vi "Image to Pixmap.vi"(8 "error in (no error)":errorcluster, 10 "image data":T1) -> (0 "error out":errorcluster, 2 "8-bit pixmap":u8[][](array[numeric]))   [LabVIEW 2016]
doc: "Takes image cluster and converts it to 8-bit pixmap. The 8-bit colors correspond to the pixmap drawn without any color input."
uses:
  <vilib>/picture/picture.llb/imagedata.ctl
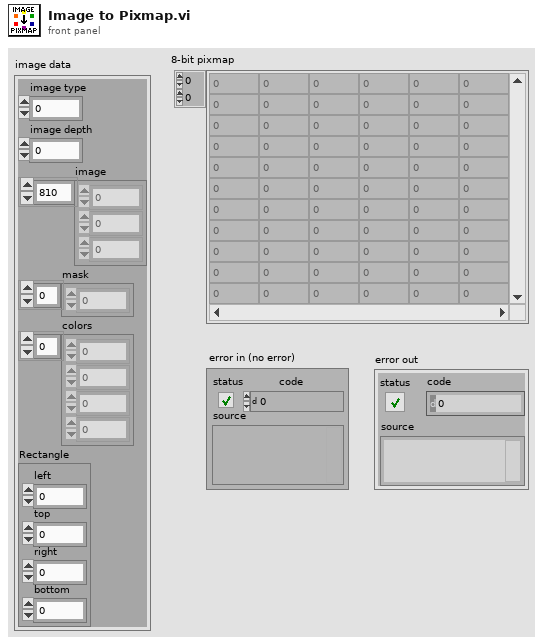
[diagram p1: front panel]
types:
  T1 = typedef "imagedata.ctl" = cluster{"image type":i32, "image depth":i32, "image":u8[], "mask":u8[], "colors":u32[], "Rectangle":cluster{"left":i16, "top":i16, "right":i16, "bottom":i16}}
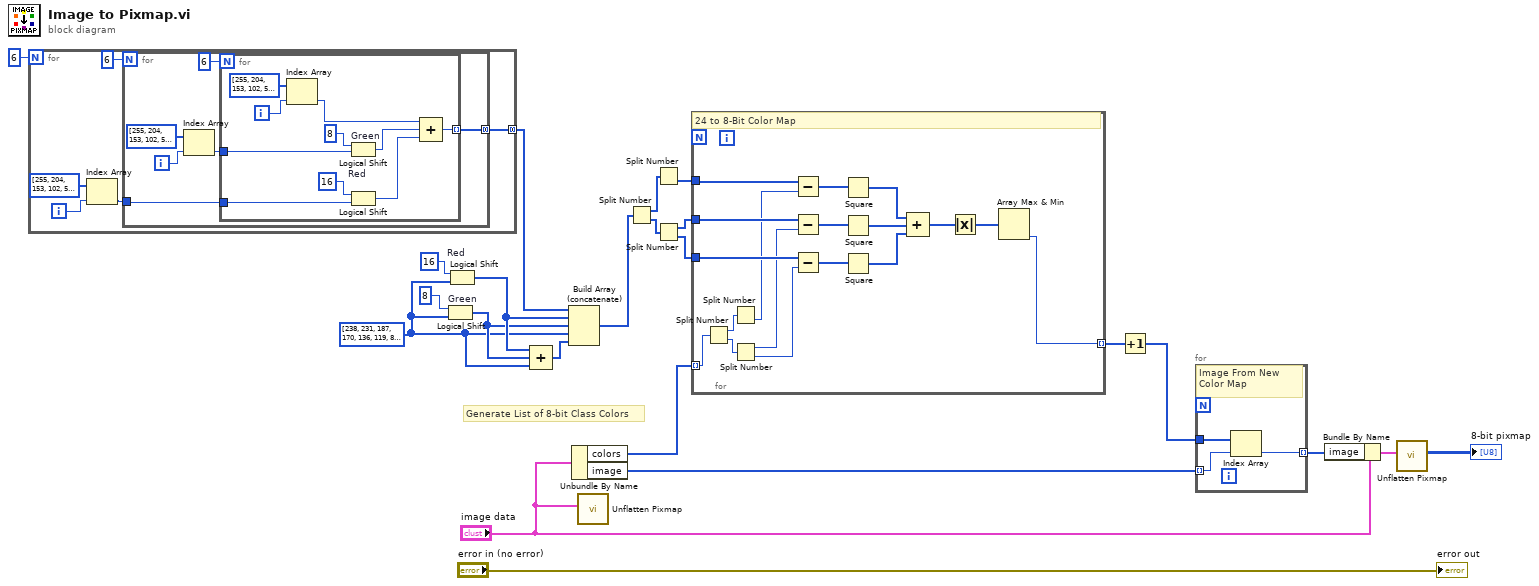
[diagram p0: block diagram]
diagram:
  w18 = u32[] [238, 231, 187, 170, 136, 119, 86, 68, 34, 17]
  # "Generate List of 8-bit Class Colors"
  n1 = for {
    N: 6 -> [_]
    tunnel: [w25] -> w16 mode=concatenating
    i -> [w27]
    n2 = Index Array(array=u32[] [255, 204, 153, 102, 51, 0], index=w27) -> (element=w26:u32)
    n3 = for {
      N: 6 -> [_]
      tunnel: w26 -> [w31]
      tunnel: [w30] -> w25 mode=concatenating
      i -> [w33]
      n4 = Index Array(array=u32[] [255, 204, 153, 102, 51, 0], index=w33) -> (element=w32:u32)
      n5 = for {
        N: 6 -> [_]
        tunnel: w32 -> [w39]
        tunnel: w31 -> [w38]
        tunnel: [w35] -> w30 mode=indexing
        i -> [w43]
        n6 = Index Array(array=u32[] [255, 204, 153, 102, 51, 0], index=w43) -> (element=w42:u32)
        n7 = Logical Shift "Green"(y=i16 8, x=w39) -> (x << y=w37:u32)
        n8 = Logical Shift "Red"(y=i16 16, x=w38) -> (x << y=w36:u32)
        n9 = Compound Arithmetic op=ADD(w42, w37, w36) -> (w35:u32)
      }
    }
  }
  n10 = Logical Shift "Green"(y=i16 8, x=w18) -> (x << y=w19:u32[])
  n11 = Logical Shift "Red"(y=i16 16, x=w18) -> (x << y=w20:u32[])
  n12 = Compound Arithmetic op=unknown(w20, w19, w18) -> (w17:u32[])
  n13 = Build Array (concatenate)(w16, w20, w19, w18, w17) -> (w9:u32[])
  n14 = Unbundle By Name("image data") -> ("colors"=w15:u32[], "image"=w14:u8[])
  n15 = call <vilib>:"Unflatten Pixmap.vi"("image data"="image data") -> ()  [unwired: 4 in, 7 out]
  n16 = Split Number(x=w9) -> (hi(x)=w10:u16[], lo(x)=w11:u16[])
  n17 = Split Number(x=w10) -> (lo(x)=w7:u8[])  [unwired: 1 out]
  n18 = Split Number(x=w11) -> (hi(x)=w6:u8[], lo(x)=w8:u8[])
  n19 = for {
    tunnel: w15 -> [w60] mode=indexing
    tunnel: w8 -> [w58]
    tunnel: w7 -> [w54]
    tunnel: w6 -> [w56]
    tunnel: [w47] -> w5 mode=indexing
    # "24 to 8-Bit Color Map"
    n20 = Split Number(x=w60) -> (hi(x)=w62:u16, lo(x)=w61:u16)
    n21 = Split Number(x=w62) -> (lo(x)=w55:u8)  [unwired: 1 out]
    n22 = Split Number(x=w61) -> (hi(x)=w57:u8, lo(x)=w59:u8)
    n23 = Subtract(x=w54, y=w55) -> (x-y=w50:i64[])
    n24 = Subtract(x=w56, y=w57) -> (x-y=w49:i64[])
    n25 = Subtract(x=w58, y=w59) -> (x-y=w48:i64[])
    n26 = Square(x=w50) -> (x^2=w53:i64[])
    n27 = Square(x=w49) -> (x^2=w52:i64[])
    n28 = Square(x=w48) -> (x^2=w51:i64[])
    n29 = Compound Arithmetic op=ADD(w53, w52, w51) -> (w45:i64[])
    n30 = Absolute Value(x=w45) -> (abs(x)=w46:i64[])
    n31 = Array Max & Min(array=w46) -> (min index (indices)=w47:i32)  [unwired: 3 out]
  }
  n32 = Increment(x=w5) -> (x+1=w2:i32[])
  n33 = for {
    tunnel: w14 -> [w65] mode=indexing
    tunnel: w2 -> [w63]
    tunnel: [w64] -> w4 mode=indexing
    # "Image From New Color Map"
    n34 = Index Array "Index Array"(array=w63, index=w65) -> (element=w64:i32)
  }
  n35 = Bundle By Name(cluster="image data", "image"=w4) -> (w13:T1)
  n36 = call <vilib>:"Unflatten Pixmap.vi"("image data"=w13) -> ("8-bit pixmap"=→"8-bit pixmap":u8[][])  [unwired: 4 in, 6 out]
  "error out" <- "error in (no error)"
